vi "LVClass_HasoData Get Compute Slopes Set.vi"(0 "HasoData in":refnum<class "HasoData.lvclass">, 11 "error in (no error)":errorcluster) -> (4 "HasoData out":refnum<class "HasoData.lvclass">, 8 "SLOPES ENGINE information":T2={"Start sub-aperture"={"X"=0, "Y"=0}, "Pupil average"=670.0, "AutoStartSub-aperture"=FALSE} {"Pupil average" min=0.0 max=1.0}, 10 "Start sub-aperture Array":T1[](array[typedef]), 12 "spot_tracker":bool, 13 "lift_algo":bool, 14 "els_algo":bool, 15 "error out":errorcluster)   [LabVIEW 2020, in "HasoData.lvclass"]
doc: "Get informations from HasoData object.\n\n<B>HasoDataIn</B> : HasoData object.\n<B>HasoDataOut</B> : HasoData object.\n<B>wavelength_nm</B> : Source wavelength (nm).\n<B>start_subpupil</B> : Start subpupil position (first element of the start_subpupil Array)\n<B>start_subpupil Array </B> : Array of coordinates of sub-pupil use to compute in multi aperture (index coordinates relative to the top-left corner of the pupil).\n<B>denoising_strength</B> : Sensitivity of spot detection (between 0 and 1). Modulates noise management\n when computing slopes on summed images.\n * 0 : Release constraint on noise to detect as much sub-pupils as possible.\n * 1 : Do not take into account the noise reduction caused by summing.\n<B>auto_start </B> : Activation of the auto start subpupil detection in case specified start subpupil is not found\n<B>spot tracker activation </B> : Spot tracker Activation during slopes computation\n<B>els algo activation </B> : Extended Light Source algorithm during slopes computation\n<B>lift algo activation </B> : LIFT algorithm during slopes computation\n\n<B>ErrorIn </B> : Error\n<B>ErrorOut </B> : Error"
uses:
  HasoData.lvclass
  SlopesEngineSetup.ctl
  Point2D.ctl
  HasoData.lvclass/HasoData.ctl
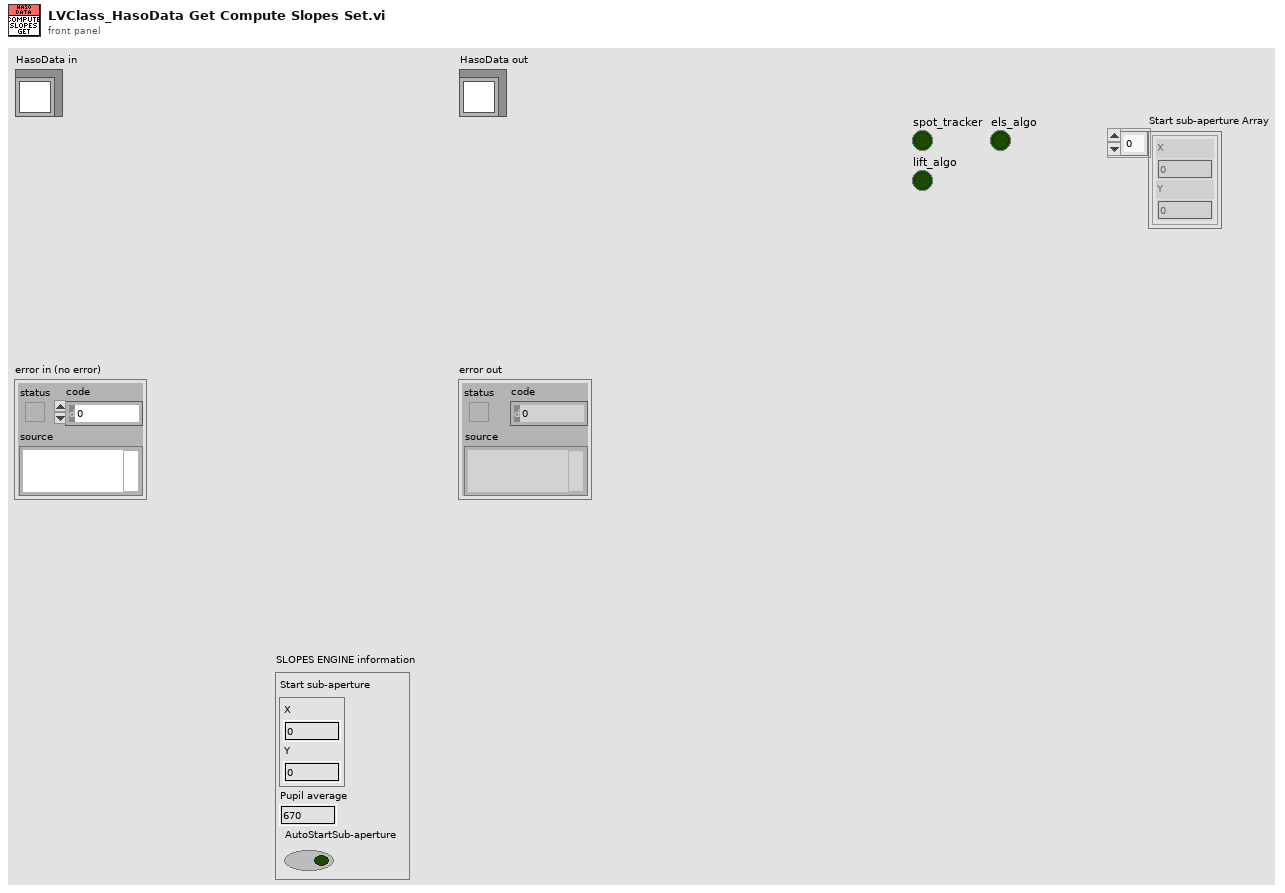
[diagram p1: front panel]
types:
  T1 = typedef "Point2D.ctl" = cluster{"X":u32, "Y":u32}
  T2 = typedef "SlopesEngineSetup.ctl" = cluster{"Start sub-aperture":T1, "Pupil average":dbl, "AutoStartSub-aperture":bool}
  T3 = typedef "ClassID.ctl" = i64
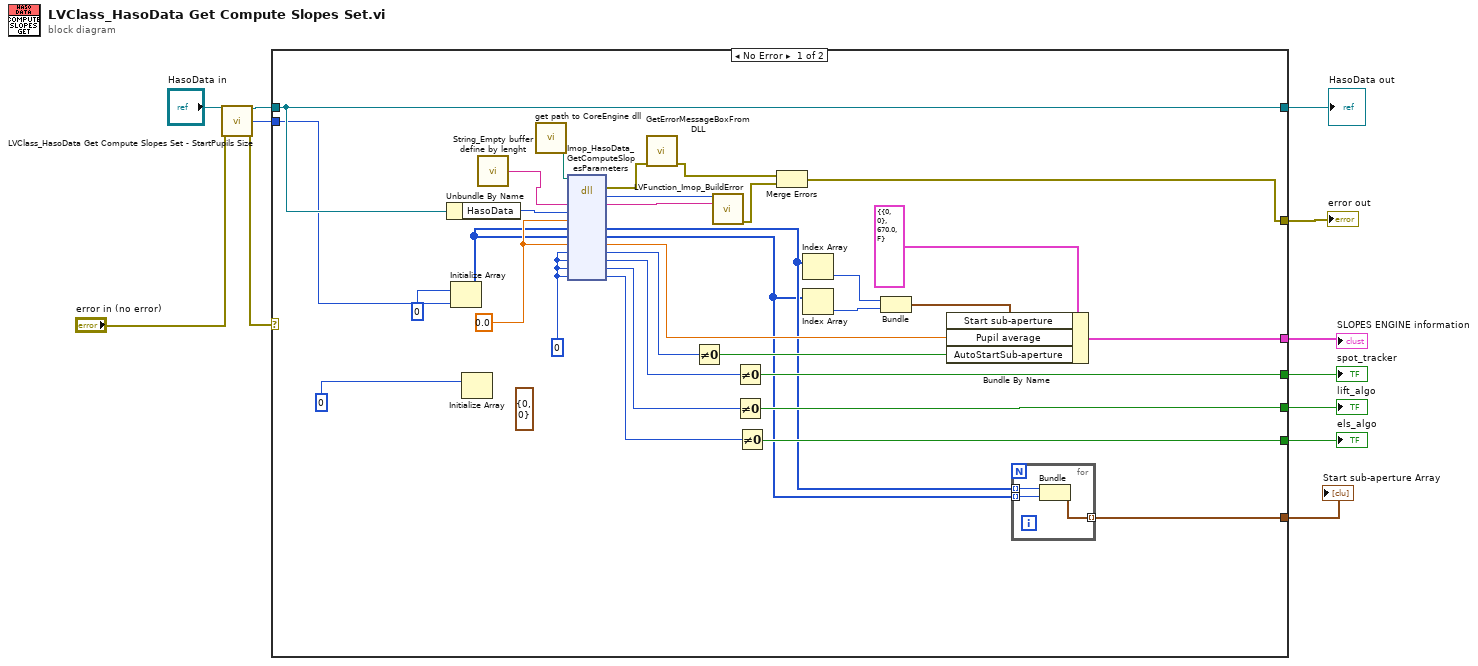
[diagram p0: block diagram]
diagram:
  n1 = call "LVClass_HasoData Get Compute Slopes Set - StartPupils Size.vi"("HasoData in"="HasoData in", "error in (no error)"="error in (no error)") -> ("HasoData out"=w5:refnum<class "HasoData.lvclass">, "Size"=w2:i32, "error out"=w3:errorcluster)  [unwired: 11 in]
  n2 = case shown="No Error" w3 {
    selector: w3 -> [_ w50]
    tunnel: [w36 w50] -> w12
    tunnel: [w41 w49] -> w11
    tunnel: w5 -> [w41 w49]
    tunnel: [w39 _] -> w10
    tunnel: [w26 _] -> w9
    tunnel: [w25 _] -> w8
    tunnel: [w24 _] -> w7
    tunnel: w2 -> [w20 _]
    tunnel: [w13 _] -> w1
    frame No Error {
      (unwired) T1 {"X"=0, "Y"=0} ("Size")
      w32 = u8 0 ("auto_start")
      w23 = 0.0 ("Pupil average")
      n3 = Unbundle By Name(w41) -> ("HasoData"=w40:T3)
      n4 = Initialize Array(u32 0 ("X"), w20) -> (w19:u32[])
      n5 = Initialize Array(u32 0 ("X")) -> ()  [unwired: 1 in, 1 out]
      n6 = call "String_Empty buffer define by lenght.vi"() -> ("Empty buffer"=w34:string)  [unwired: 1 in]
      n7 = call "get path to CoreEngine dll.vi"() -> ("path to wavekit library"=w43:path)  [unwired: 14 in, 1 out]
      n8 = dll-call lib="D:/soft/HASO_v3/SVN_trunk/ImOpCoreEngine4_LV2011/DLLs/c_interface_vc100.dll" fn="Imop_HasoData_GetComputeSlopesParameters"(path in=w43, "message"=w34, "HasoData"=w40, "wavelength_nm"=w23, "StartSubPupil_X"=w19, "StartSubPupil_Y"=w19, "Pupil average"=w23, "auto_start"=w32, "spot_tracker"=w32, "lift_algo"=w32, "els_algo"=w32) -> (error out=w42:errorcluster, "return type"=w45:i32, "message"=w44:string, "StartSubPupil_X"=w18:i32[], "StartSubPupil_Y"=w17:i32[], "Pupil average"=w35:dbl, "auto_start"=w31:u8, "spot_tracker"=w30:u8, "lift_algo"=w29:u8, "els_algo"=w28:u8)  [unwired: 4 in, 1 out]
      n9 = call "GetErrorMessageBoxFromDLL.vi"("error IN"=w42) -> ("error OUT"=w38:errorcluster)  [unwired: 10 in]
      n10 = Not Equal To 0?(x=w31) -> (x != 0?=w27:bool)
      n11 = call "LVFunction_Imop_BuildError.vi"("code"=w45, "String to Prepend to source (\"\")"=w44) -> ("error out"=w37:errorcluster)  [unwired: 13 in]
      n12 = Not Equal To 0?(x=w30) -> (x != 0?=w26:bool)
      n13 = Not Equal To 0?(x=w29) -> (x != 0?=w25:bool)
      n14 = Not Equal To 0?(x=w28) -> (x != 0?=w24:bool)
      n15 = Merge Errors(w38, w37) -> (w36:errorcluster)
      n16 = Index Array(array=w18) -> (element=w16:i32)  [unwired: 1 in]
      n17 = Index Array(array=w17) -> (element=w15:i32)  [unwired: 1 in]
      n18 = Bundle(w16, w15) -> (w14:cluster{i32, i32})  [unwired: 1 in]
      n19 = Bundle By Name(cluster=T2 {"Start sub-aperture"={"X"=0, "Y"=0}, "Pupil average"=670.0, "AutoStartSub-aperture"=FALSE} ("SLOPES ENGINE information"), "Start sub-aperture"=w14, "Pupil average"=w35, "AutoStartSub-aperture"=w27) -> (w39:T2)
      n20 = for {
        tunnel: w18 -> [w48] mode=indexing
        tunnel: w17 -> [w47] mode=indexing
        tunnel: [w46] -> w13 mode=indexing
        n21 = Bundle(w48, w47) -> (w46:cluster{i32, i32})  [unwired: 1 in]
      }
    }
    frame Error {
    }
  }
  "error out" <- w12
  "HasoData out" <- w11
  "SLOPES ENGINE information" <- w10
  "spot_tracker" <- w9
  "lift_algo" <- w8
  "els_algo" <- w7
  "Start sub-aperture Array" <- w1
